vi "I2C Comms.vi"() -> (0 "error out":errorcluster, 3 "I2CDevRef out":T1 {"Device Address" format="%.0x"})   [LabVIEW 2013]
uses:
  <vilib>/Rock Robotics/WPI/I2C/WPI_I2CDevRef.ctl
  <vilib>/Rock Robotics/SystemInterfaces/Typedef/FPGA_TypedefDigitalModule.ctl
  Pressure State.ctl
  Drivetrain/DT Mode.ctl
  Robot Global Data.vi
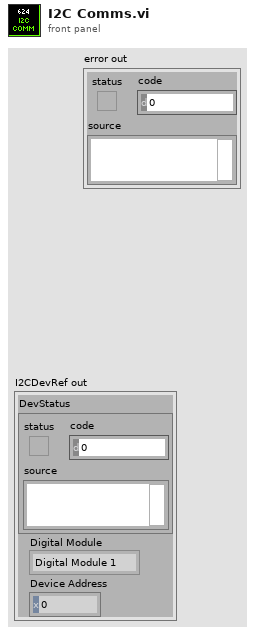
[diagram p1: front panel]
types:
  T1 = typedef "WPI_I2CDevRef.ctl" = cluster{"DevStatus":errorcluster, "Digital Module":T2, "Device Address":u8}
  T2 = typedef "FPGA_TypedefDigitalModule.ctl" = enum16{"Digital Module 1", "Digital Module 2"}
  T3 = typedef "DT Mode.ctl" = enum16{"Manual", "Gyro Steer", "Distance Drive", "Fieldcentric", "Roll Maneuver", "Alt Roll Maneuver"}
  T4 = typedef "Pressure State.ctl" = enum16{"Full", "Low", "Empty"}
  T5 = typedef "Shooter Status.ctl" = cluster{"Shooter Ready":bool, "Add":bool, "Punch":bool, "Release":bool, "Trigger":bool, "High":bool, "State":T6}
  T6 = typedef "Shooter State.ctl" = enum16{"Wait", "Fill Piston", "Lift Halo", "Trigger", "Reset", "Soft Release", "Soft Unpin", "Soft Refill", "Soft Shoot", "Toss Prep", "Toss Release"}
  T7 = typedef "Drivetrain Status.ctl" = cluster{"Mode":T3, "X":dbl, "Y":dbl, "Steer":dbl, "Low Gear":bool, "Omni":bool}
  T8 = typedef "WPI_DriverStationRobotMode2.ctl" = enum16{"Autonomous Disabled", "Autonomous Enabled", "Teleop Disabled", "Teleop Enabled", "Timeout", "Finish", "Test Disabled", "Test Enabled"}
  T9 = typedef "WPI_DriverStationAllianceInfo.ctl" = enum16{"Red", "Blue", "Invalid"}
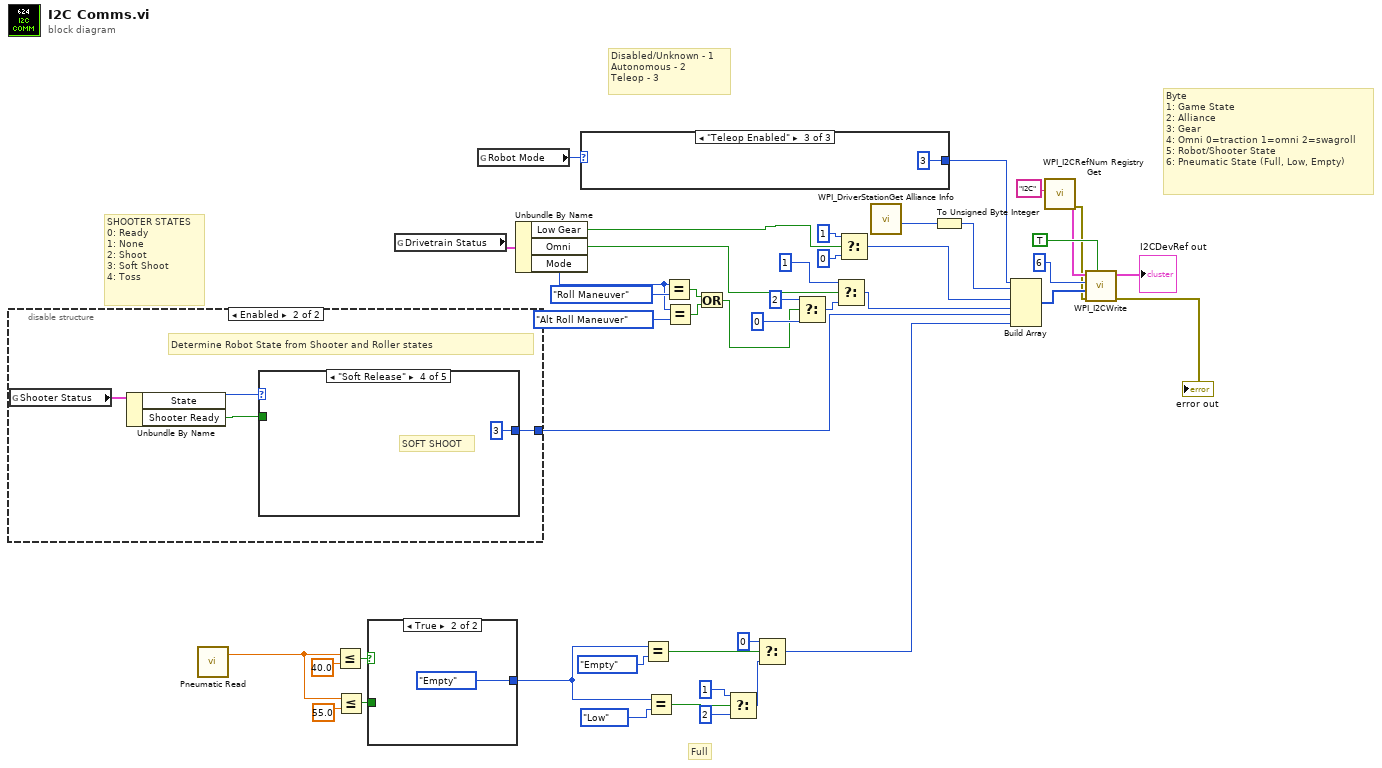
[diagram p0: block diagram]
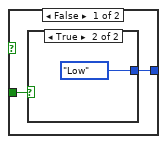
[diagram p2: hidden frame]
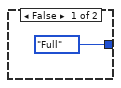
[diagram p3: hidden frame]
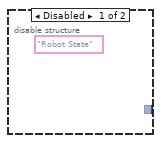
[diagram p4: hidden frame]
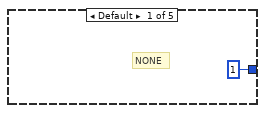
[diagram p5: hidden frame]
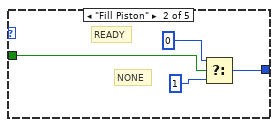
[diagram p6: hidden frame]
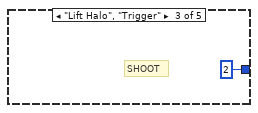
[diagram p7: hidden frame]
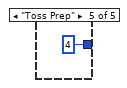
[diagram p8: hidden frame]
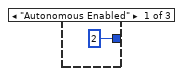
[diagram p9: hidden frame]
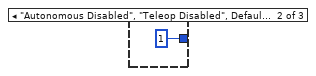
[diagram p10: hidden frame]
diagram:
  # "SHOOTER STATES\n0: Ready\n1: None\n2: Shoot\n3: Soft Shoot\n4: Toss"
  # "Full"
  # "Byte\n1: Game State\n2: Alliance\n3: Gear\n4: Omni 0=traction 1=omni 2=swagroll\n5: Robot/Shooter State\n6: Pneumatic State (Full, Low, Empty)"
  # "Disabled/Unknown - 1\nAutonomous - 2\nTeleop - 3"
  n1 = disable-structure shown="Enabled" {
    disable-tunnel: [w46 w51] -> w1
    frame Disabled {
      w47 = "Robot State" ("Name")
    }
    frame Enabled {
      # "Determine Robot State from Shooter and Roller states"
      n2 = global read "Robot Global Data.vi" "Shooter Status"() -> (w50:T5)
      n3 = Unbundle By Name(w50) -> ("State"=w49:T6, "Shooter Ready"=w48:bool)
      n4 = case shown="\"Soft Release\"" w49 {
        tunnel: [1 w56 2 3 4] -> w51
        tunnel: w48 -> [_ w55 _ _ _]
        frame Default {
          # "NONE"
        }
        frame "Fill Piston" {
          # "NONE"
          # "READY"
          n5 = Select(t=0, s=w55, f=1) -> (s? t:f=w56:i32)
        }
        frame "Lift Halo", "Trigger" {
          # "SHOOT"
        }
        frame "Soft Release" {
          # "SOFT SHOOT"
        }
        frame "Toss Prep" {
        }
      }
    }
  }
  n6 = call "Pneumatic Read.vi"() -> ("Line"=w30:dbl)  [unwired: 2 in, 1 out]
  n7 = Less Or Equal?(x=w30, y=40.0) -> (x <= y?=w29:bool)
  n8 = Less Or Equal?(x=w30, y=55.0) -> (x <= y?=w28:bool)
  n9 = case shown="True" w29 {
    tunnel: w28 -> [w61 _]
    tunnel: [w60 Pressure_State."Empty"] -> w19
    frame False {
      n10 = case shown="True" w61 {
        tunnel: [Pressure_State."Full" Pressure_State."Low"] -> w60
        frame False {
        }
        frame True {
        }
      }
    }
    frame True {
    }
  }
  n11 = global read "Robot Global Data.vi" "Drivetrain Status"() -> (w13:T7)
  n12 = global read "Robot Global Data.vi" "Robot Mode"() -> (w43:T8)
  n13 = Unbundle By Name(w13) -> ("Low Gear"=w12:bool, "Omni"=w11:bool, "Mode"=w9:T3)
  n14 = case shown="\"Teleop Enabled\"" w43 {
    tunnel: [u8 2 u8 1 u8 3] -> w45
    frame "Autonomous Enabled" {
    }
    frame "Autonomous Disabled", "Teleop Disabled", Default {
    }
    frame "Teleop Enabled" {
    }
  }
  n15 = Equal?(x=w19, y=Pressure_State."Empty") -> (x = y?=w26:bool)
  n16 = Equal?(x=w19, y=Pressure_State."Low") -> (x = y?=w23:bool)
  n17 = Equal?(x=w9, y=DT_Mode."Roll Maneuver") -> (x = y?=w7:bool)
  n18 = Equal?(x=w9, y=DT_Mode."Alt Roll Maneuver") -> (x = y?=w6:bool)
  n19 = Or(x=w7, y=w6) -> (x .or. y?=w3:bool)
  n20 = Select(t=u8 1, s=w23, f=u8 2) -> (s? t:f=w21:u8)
  n21 = Select(t=u8 0, s=w26, f=w21) -> (s? t:f=w20:u8)
  n22 = Select(t=u8 2, s=w3, f=u8 0) -> (s? t:f=w2:u8)
  n23 = Select(t=u8 1, s=w11, f=w2) -> (s? t:f=w33:u8)
  n24 = Select(t=u8 1 ("I2CRegister"), s=w12, f=u8 0) -> (s? t:f=w34:u8)
  n25 = call <vilib>:"WPI_DriverStationGet Alliance Info.vi"() -> ("Alliance"=w41:T9)  [unwired: 10 in, 1 out]
  n26 = To Unsigned Byte Integer(number=w41) -> (unsigned 8bit integer=w40:u8)
  n27 = Build Array(w45, w40, w34, w33, w1, w20) -> (w44:i32[])
  n28 = call <vilib>:"WPI_I2CRefNum Registry Get.vi"("refnum name"="I2C") -> ("error out"=w15:errorcluster, "I2CDevRef"=w16:T1)  [unwired: 9 in]
  n29 = call <vilib>:"WPI_I2CWrite.vi"("CompatibilityMode"=TRUE, "error in (no error)"=w15, "I2CDataToSend"=w44, "I2CRegister"=u8 6, "I2CDevRef"=w16) -> ("error out"=→"error out":errorcluster, "I2CDevRef"=→"I2CDevRef out":T1)  [unwired: 5 in]
